vi "Z Aux Direct Move Aout.vi"(8 "error in (no error)":errorcluster caption="错误输入（无错误）", 9 "fvalue":sgl, 10 "ioutnum":i32, 11 "handle":u32) -> (0 "error out":errorcluster caption="错误输出", 2 "function return":i32, 3 "handle out":u32)   [LabVIEW 2015, in "zauxdll.lvlib"]
doc: "int32 __stdcall ZAux_Direct_MoveAout(ZMC_HANDLE handle, int ioutnum, float fvalue);"
uses:
  zauxdll.lvlib
  Radar - 2015 32bit_autoqueue_angle_0319/zauxdll-2014/zauxdll.dll
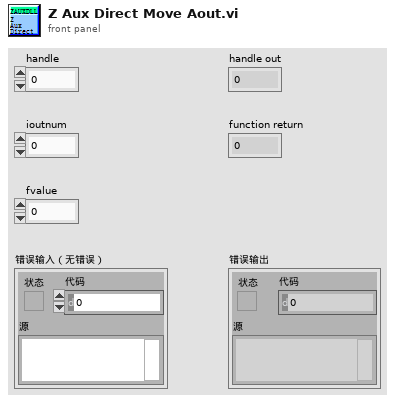
[diagram p1: front panel]
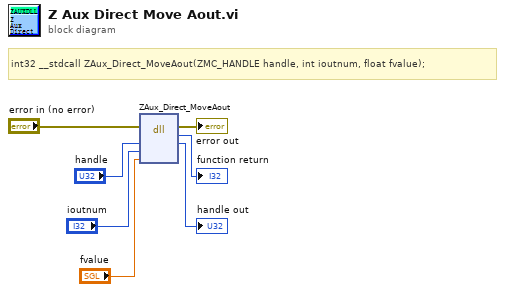
[diagram p0: block diagram]
diagram:
  # "int32 __stdcall ZAux_Direct_MoveAout(ZMC_HANDLE handle, int ioutnum, float fvalue);"
  n1 = dll-call lib="D:/vicomm case/cub/0717/Radar - 2015 32bit_autoqueue_angle_0319/zauxdll-2014/zauxdll.*" fn="ZAux_Direct_MoveAout"(error in="error in (no error)", "handle"="handle", "ioutnum"="ioutnum", "fvalue"="fvalue") -> (error out=→"error out":errorcluster, →"function return":i32, "handle"=→"handle out":u32)  [unwired: 4 in, 1 out]
